vi "NT Read With Override.vi"(9 "Overide Numeric":dbl, 11 "Name":string="Numeric") -> (3 "Numeric":dbl)   [LabVIEW 2016]
doc: "This VI is used for overiding the dashboard. When the Overide NT Boolean is true it sends through the Overide Numeric as opposed to the NTRead.\n\nCreated by Team 4130 for use in the 2016-2017 FRC season"
uses:
  <vilib>/Rock Robotics/Network Tables/NT Read Number.vi
  <vilib>/Rock Robotics/Network Tables/NT Read Boolean.vi
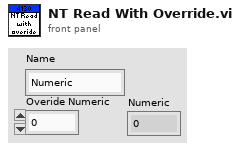
[diagram p1: front panel]
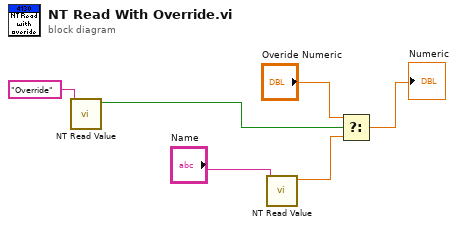
[diagram p0: block diagram]
diagram:
  n1 = call-poly <vilib>:"NT Read Value.vi"("Name"="Override") -> ("Boolean"=w3:bool)  [unwired: 9 in, 1 out]
  n2 = call-poly <vilib>:"NT Read Value.vi"("Name"="Name") -> ("Numeric"=w5:dbl)  [unwired: 9 in, 1 out]
  n3 = Select(t="Overide Numeric", s=w3, f=w5) -> (s? t:f=→"Numeric":dbl)
